vi "Rotate 3D object.vi"() -> ()   [LabVIEW 2014]
uses:
  <vilib>/LabVIEW Hacker/LINX/Private/Type Defs/User Platform.ctl
  <vilib>/picture/3D Picture Control/Object/Create Object (name).vi
  <vilib>/picture/3D Picture Control/NI_3D Picture Control.lvlib
  <vilib>/LabVIEW Hacker/LINX/LVH-LINX.lvlib
panel:
  out "Mag-Filtered":T1
  out "Roll Pitch Yaw":T1
  in  "Chip":u16(ring)=2 items=["LSM6DS1", "LSM6DS3", "ADXL345"]
  in  "Serial Port":refnum<visa-resource-name>
  out "Device Name":string
  out "Error Out":errorcluster
  out "G-Filtered":T1
  in  "alpha":dbl=0.5 format="%#_13g"
  in  "stop":bool
  out "3D Picture":refnum<vi>(3d-picture)
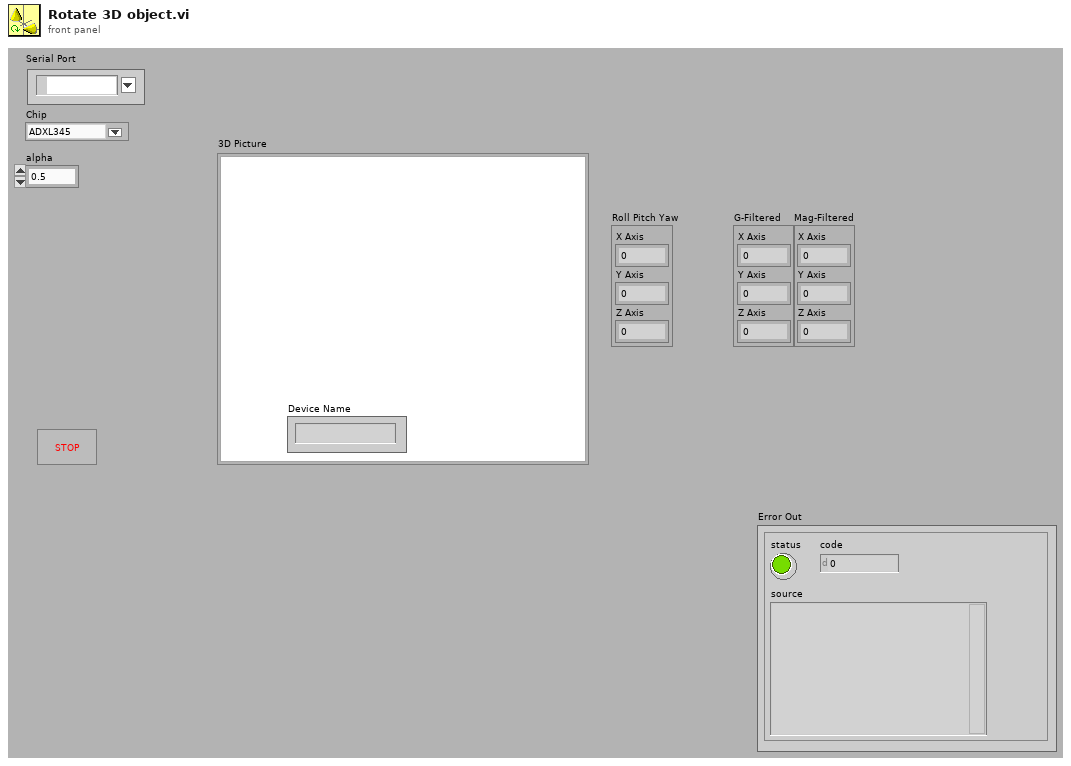
[diagram p1: front panel]
types:
  T1 = cluster{"X Axis":dbl, "Y Axis":dbl, "Z Axis":dbl}
  T2 = typedef "LVH-LINX.lvlib/User Platform.ctl" = enum16{"Default", "LINX", "myRIO"}
  T3 = typedef "LVH-LINX.lvlib/LINX Ref.ctl" = cluster{"Platform":T4, "Interface":T5, "LINX Device Config":T6}
  T4 = typedef "LVH-LINX.lvlib/Platform.ctl" = enum16{"LINX", "myRIO"}
  T5 = typedef "LVH-LINX.lvlib/Interface.ctl" = enum16{"Serial", "TCP"}
  T6 = typedef "LVH-LINX.lvlib/Device.lvlib/LINX Device Config.ctl" = cluster{"Interface":T5, "COM Port":refnum<visa-resource-name>, "TCP Configuration":T7, "Device Family":T8, "Device ID":u8, "Device Name":string, "TCP Ref":refnum<k5>}
  T7 = typedef "LVH-LINX.lvlib/Device.lvlib/TCP Config.ctl" = cluster{"IP Address":string, "Port":u16}
  T8 = typedef "LVH-LINX.lvlib/Device Family.ctl" = enum8{"National Instruments", "Digilent", "Arduino"}
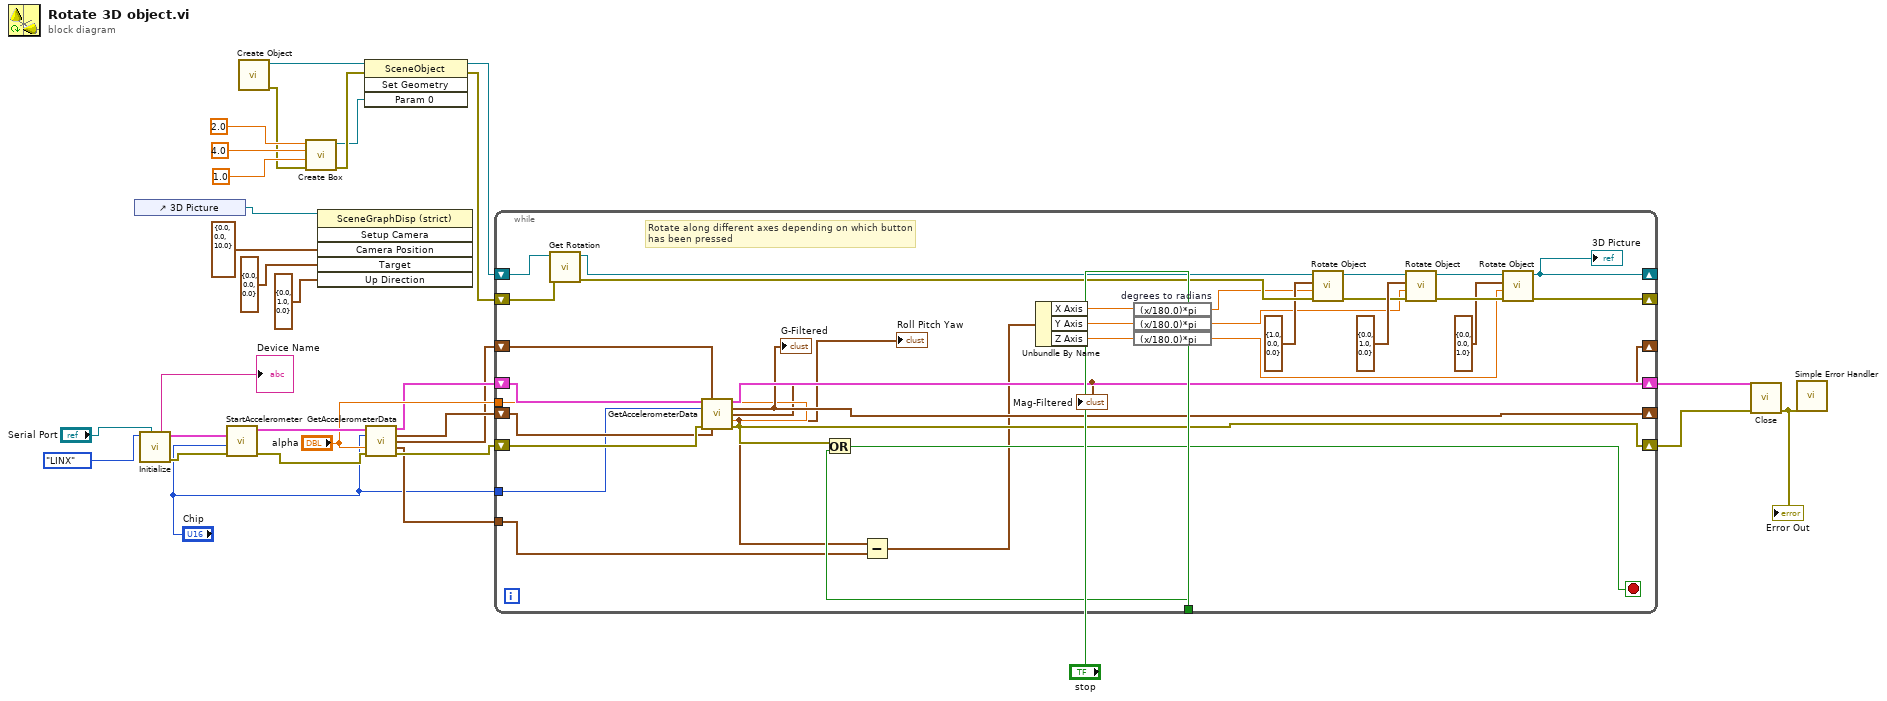
[diagram p0: block diagram]
diagram:
  n1 = control-ref of="3D Picture"() -> (w19:refnum<vi>)
  n2 = call <vilib>:"Initialize.vi"("Serial Port"="Serial Port", "Platform"=User_Platform."LINX") -> ("Error Out"=w10:errorcluster, "Device Name"=→"Device Name":string, "LINX Ref"=w11:T3)  [unwired: 7 in]
  n3 = call "StartAccelerometer.vi"("Error In"=w10, "Chip"="Chip", "LINX Resource"=w11) -> ("Error Out"=w8:errorcluster, "LINX Resource"=w9:T3)  [unwired: 3 in]
  n4 = call-poly <vilib>:"Create Object.vi"() -> ("error out"=w22:errorcluster, "Scene:New Object"=w28:refnum<vi>)  [unwired: 10 in]
  n5 = call <vilib>:"Create Box.vi"("error in (no error)"=w22, "Length Z"=sgl 1.0, "Length Y"=sgl 4.0, "Length X"=sgl 2.0) -> ("error out"=w21:errorcluster, "New Box Refnum"=w20:refnum<vi>)  [unwired: 6 in]
  n6 = invoke on="Invoke Node" class="SceneGraphDisp (strict)" method="Setup Camera"(reference=w19, "Camera Position"=cluster{"X":sgl, "Y":sgl, "Z":sgl} {"X"=0.0, "Y"=0.0, "Z"=10.0}, "Target"=cluster{"X":sgl, "Y":sgl, "Z":sgl} {"X"=0.0, "Y"=0.0, "Z"=0.0}, "Up Direction"=cluster{"X":sgl, "Y":sgl, "Z":sgl} {"X"=0.0, "Y"=1.0, "Z"=0.0}) -> ()  [unwired: 2 in, 6 out]
  n7 = invoke class="SceneObject" method="Set Geometry"(reference=w28, error in=w21, "Param 0"=w20) -> (reference out=w27:refnum<vi>, error out=w26:errorcluster)  [unwired: 1 in, 2 out]
  n8 = call "GetAccelerometerData.vi"("LINX Resource"=w9, "Chip"="Chip", "alpha"="alpha", "Error In"=w8) -> ("LINX Resource"=w5:T3, "G-Filtered"=w4:T1, "Mag-Filtered"=w3:T1, "Roll Pitch Yaw"=w2:T1, "Error Out"=w7:errorcluster)  [unwired: 7 in]
  n9 = while {
    shift-right: [w34] -> _
    shift-left: w27 -> [w65]
    shift-right: [w39] -> _
    shift-left: w26 -> [w64]
    tunnel: "stop" -> [w59]
    shift-right: [w58] -> w16
    shift-left: w7 -> [w57]
    shift-right: [w56] -> _
    shift-left: w4 -> [w55]
    shift-right: [w60] -> w15
    shift-left: w5 -> [w54]
    tunnel: "alpha" -> [w44]
    shift-right: [w32] -> _
    shift-left: w3 -> [w43]
    tunnel: "Chip" -> [w33]
    tunnel: w2 -> [w49]
    stop <- w61 stop-if-true
    # "Rotate along different axes depending on which button\nhas been pressed"
    n10 = call <vilib>:"Get Rotation.vi"("error in (no error)"=w64, "Scene Object"=w65) -> ("error out"=w62:errorcluster, "Scene Object"=w63:refnum<vi>)  [unwired: 6 in, 2 out]
    n11 = call "GetAccelerometerData.vi"("LINX Resource"=w54, "input Mag"=w43, "Chip"=w33, "alpha"=w44, "Error In"=w57, "input Gs"=w55) -> ("LINX Resource"=w60:T3, "G-Filtered"=w56:T1, "Mag-Filtered"=w32:T1, "Roll Pitch Yaw"=w42:T1, "Error Out"=w58:errorcluster)  [unwired: 5 in]
    "G-Filtered" <- w56
    "Roll Pitch Yaw" <- w42
    "Mag-Filtered" <- w32
    n12 = Or(x=w58, y=w59) -> (x .or. y?=w61:bool)
    n13 = Subtract(x=w42, y=w49) -> (x-y=w41:T1)
    n14 = Unbundle By Name(w41) -> ("X Axis"=w48:dbl, "Y Axis"=w46:dbl, "Z Axis"=w36:dbl)
    n15 = expression code="(x/180.0)*pi" "degrees to radians"(w48) -> (w47:dbl)
    n16 = expression code="(x/180.0)*pi" ("degrees to radians")(w46) -> (w45:dbl)
    n17 = expression code="(x/180.0)*pi" ("degrees to radians")(w36) -> (w35:dbl)
    n18 = call <vilib>:"Rotate Object.vi"("error in (no error)"=w62, "Angle"=w47, "Axis"=cluster{"X":sgl, "Y":sgl, "Z":sgl} {"X"=1.0, "Y"=0.0, "Z"=0.0}, "Scene.Object In"=w63) -> ("error out"=w51:errorcluster, "Scene.Object Out"=w53:refnum<vi>)  [unwired: 6 in]
    n19 = call <vilib>:"Rotate Object.vi"("error in (no error)"=w51, "Angle"=w45, "Axis"=cluster{"X":sgl, "Y":sgl, "Z":sgl} {"X"=0.0, "Y"=1.0, "Z"=0.0}, "Scene.Object In"=w53) -> ("error out"=w38:errorcluster, "Scene.Object Out"=w40:refnum<vi>)  [unwired: 6 in]
    n20 = call <vilib>:"Rotate Object.vi"("error in (no error)"=w38, "Angle"=w35, "Axis"=cluster{"X":sgl, "Y":sgl, "Z":sgl} {"X"=0.0, "Y"=0.0, "Z"=1.0}, "Scene.Object In"=w40) -> ("error out"=w39:errorcluster, "Scene.Object Out"=w34:refnum<vi>)  [unwired: 6 in]
    "3D Picture" <- w34
  }
  n21 = call <vilib>:"Close.vi"("Error In"=w16, "LINX Resource"=w15) -> ("Error Out"=w17:errorcluster)  [unwired: 8 in, 1 out]
  "Error Out" <- w17
  n22 = call <vilib>:"Simple Error Handler.vi"("error in (no error)"=w17) -> ()  [unwired: 4 in, 5 out]
